vi "Initialize.vi"(7 "Serial Configuration":T1={"Baud Rate"=115200, "Parity"=0, "Data Bits"=8, "Stop Bits"=10, "Flow Control"=0} {"Flow Control" items=["None", "XON/XOFF", "RTS/CTS", "XON/XOFF & RTS/CTS", "DTR/DSR", "XON/XOFF & DTR/DSR"]; "Stop Bits" items=["1.0"=10, "1.5"=15, "2.0"=20]; "Data Bits" items=["7"=7, "8"=8]; "Parity" items=["None", "Odd", "Even", "Mark", "Space"]; "Baud Rate" items=["300"=300, "600"=600, "1200"=1200, "2400"=2400, "4800"=4800, "9600"=9600, "19200"=19200]}, 8 "error in (no error)":errorcluster, 10 "ID Query (True)":bool=TRUE, 11 "VISA resource name":refnum<visa-resource-name>) -> (0 "error out":errorcluster, 3 "VISA resource name out":refnum<visa-resource-name>)   [LabVIEW 2012, in "Roboteq.lvlib"]
doc: "Establishes communication with the sensor and optionally performs a sensor identification query. Therefore, call this VI before calling other sensor driver VIs for this sensor. Generally, you need to call the Initialize VI only once at the beginning of an application."
uses:
  Roboteq.lvlib
panel:
  out "read buffer 2":string
  out "Session Out":refnum<visa-resource-name>
  out "error out 3":errorcluster {"code" format="%.0x"}
  out "token":string
  in  "error in":errorcluster {"code" format="%.0x"}
  in  "Session In":refnum<visa-resource-name>="COM7"
  out "error out 2":errorcluster
  out "read buffer":string
  # "(c) 2010 National Instruments.  ALL RIGHTS RESERVED."
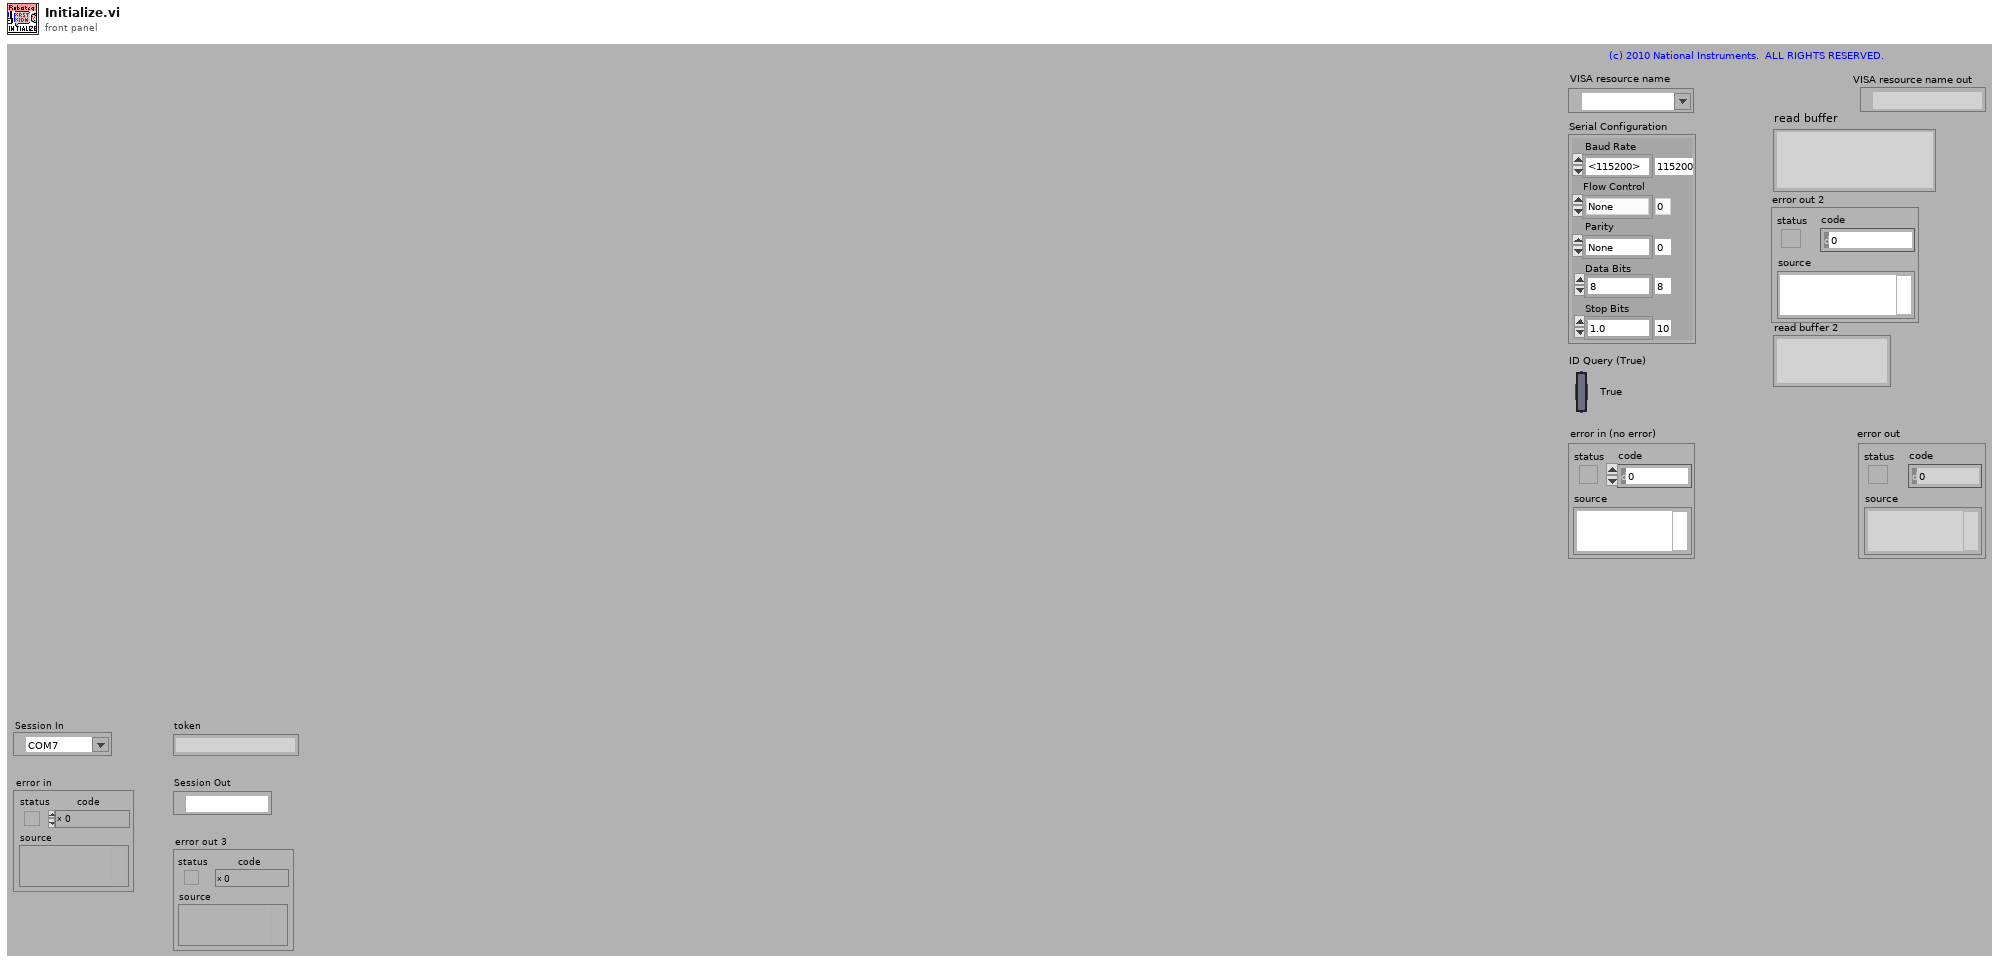
[diagram p1: front panel]
types:
  T1 = cluster{"Baud Rate":u32, "Parity":u16, "Data Bits":u16, "Stop Bits":u16, "Flow Control":u16}
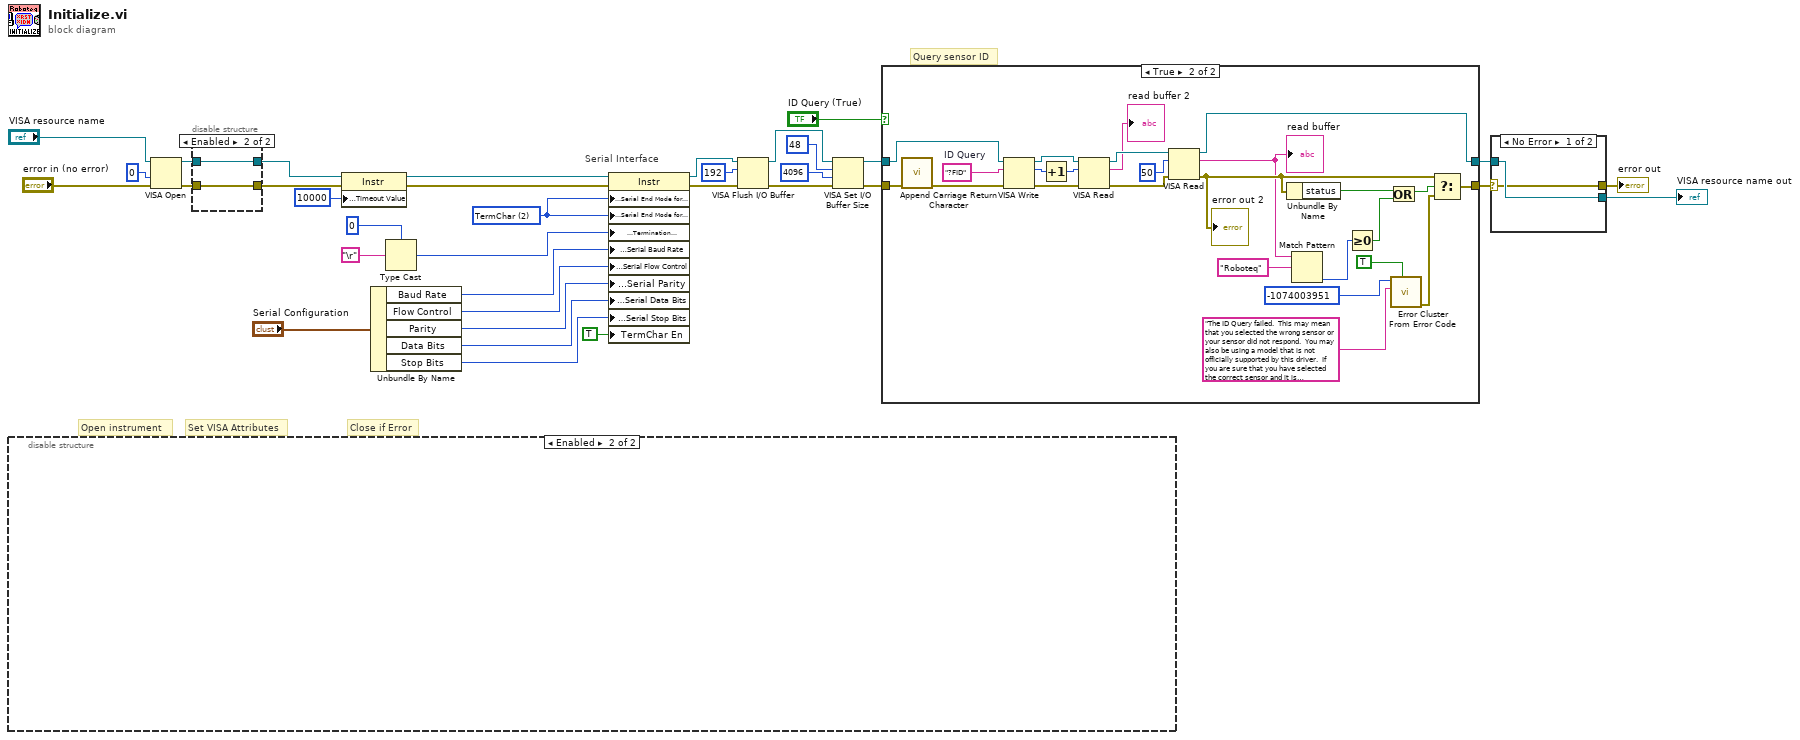
[diagram p0: block diagram]
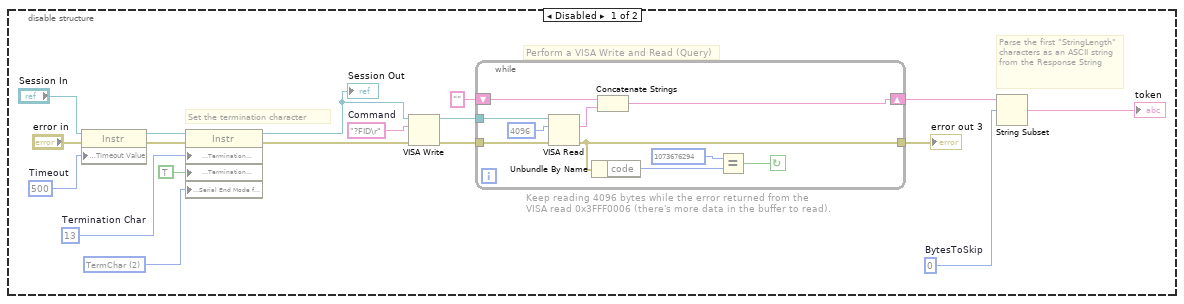
[diagram p2: hidden frame]
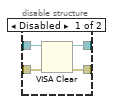
[diagram p3: hidden frame]
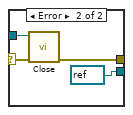
[diagram p4: hidden frame]
diagram:
  w10 = u16 2 items=["None", "LastBit", "TermChar"] ("Serial Settings:Serial End Mode for Reads")
  # "Serial Interface"
  # "Set VISA Attributes"
  # "Close if Error"
  # "Query sensor ID"
  # "Open instrument"
  n1 = disable-structure shown="Enabled" {
    frame Disabled {
      w37 = 0  # BytesToSkip
      w40 = "?FID\r"  # Command
      w45 = u16 2 items=["None", "LastBit", "TermChar"] ("ASRLEndIn")
      w48 = u8 13  # Termination Char
      w53 = u32 500  # Timeout
      # "Parse the first \"StringLength\" characters as an ASCII string from the Response String"
      # "Perform a VISA Write and Read (Query)"
      # "Keep reading 4096 bytes while the error returned from the\nVISA read 0x3FFF0006 (there's more data in the buffer to read)."
      # "Set the termination character"
      n2 = property class="Instr"(reference="Session In", error in="error in", "General Settings:Timeout Value"=w53) -> (reference out=w47:refnum<visa-resource-name>, error out=w50:errorcluster)
      n3 = property class="Instr"(reference=w47, error in=w50, "Message Based Settings:Termination Character"=w48, "Message Based Settings:Termination Character Enable"=TRUE ("enable"), "Serial Settings:Serial End Mode for Reads"=w45) -> (reference out=w36:refnum<visa-resource-name>, error out=w49:errorcluster)
      "Session Out" <- w36
      n4 = VISA Write(VISA resource name=w36, write buffer=w40, error in (no error)=w49) -> (VISA resource name out=w44:refnum<visa-resource-name>, error out=w43:errorcluster)  [unwired: 1 out]
      n5 = while {
        tunnel: w44 -> [w60]
        shift-right: [w54] -> w38
        shift-left: "" -> [w59]
        tunnel: w43 -> [w57]
        tunnel: [w56] -> w42
        stop <- w55 continue-if-true
        n6 = VISA Read(VISA resource name=w60, byte count=u32 4096 ("byte count (0)"), error in (no error)=w57) -> (read buffer=w58:string, error out=w56:errorcluster)  [unwired: 2 out]
        n7 = Unbundle By Name(w56) -> ("code"=w62:i32)
        n8 = Concatenate Strings(w59, w58) -> (w54:string)
        n9 = Equal?(x=1073676294, y=w62) -> (x = y?=w55:bool)
      }
      "error out 3" <- w42
      n10 = String Subset(string=w38, offset (0)=w37) -> (substring=→"token":string)  [unwired: 1 out]
    }
    frame Enabled {
    }
  }
  n11 = VISA Open(access mode=u32 0, error in (no error)="error in (no error)", VISA resource name="VISA resource name") -> (VISA resource name=w26:refnum<visa-resource-name>, error out=w25:errorcluster)  [unwired: 2 in]
  n12 = disable-structure shown="Enabled" {
    disable-tunnel: w26 -> [w67 w69]
    disable-tunnel: w25 -> [w66 w68]
    disable-tunnel: [w65 w69] -> w24
    disable-tunnel: [w64 w68] -> w23
    frame Disabled {
      n13 = VISA Clear(VISA resource name=w67, error in (no error)=w66) -> (VISA resource name out=w65:refnum<visa-resource-name>, error out=w64:errorcluster)
    }
    frame Enabled {
    }
  }
  n14 = property class="Instr"(reference=w24, error in=w23, "General Settings:Timeout Value"=u32 10000) -> (reference out=w29:refnum<visa-resource-name>, error out=w28:errorcluster)
  n15 = Unbundle By Name("Serial Configuration") -> ("Baud Rate"=w8:u32, "Flow Control"=w4:u16, "Parity"=w6:u16, "Data Bits"=w7:u16, "Stop Bits"=w3:u16)
  n16 = Type Cast(type=u8 0, x="\r") -> (*(type *) &x=w9:u8)
  n17 = property class="Instr"(reference=w29, error in=w28, "Serial Settings:Serial End Mode for Reads"=w10, "Serial Settings:Serial End Mode for Writes"=w10, "Message Based Settings:Termination Character"=w9, "Serial Settings:Serial Baud Rate"=w8, "Serial Settings:Serial Flow Control"=w4, "Serial Settings:Serial Parity"=w6, "Serial Settings:Serial Data Bits"=w7, "Serial Settings:Serial Stop Bits"=w3, "TermChar En"=TRUE) -> (reference out=w16:refnum<visa-resource-name>, error out=w18:errorcluster)
  n18 = VISA Flush I/O Buffer(VISA resource name=w16, mask (16)=u16 192, error in (no error)=w18) -> (VISA resource name out=w19:refnum<visa-resource-name>, error out=w17:errorcluster)
  n19 = VISA Set I/O Buffer Size(VISA resource name=w19, mask (16)=u16 48, size (4096)=u32 4096 ("size (0)"), error in (no error)=w17) -> (VISA resource name out=w31:refnum<visa-resource-name>, error out=w30:errorcluster)
  n20 = case shown="True" "ID Query (True)" {
    tunnel: [w70 w96] -> w1
    tunnel: [w71 w82] -> w20
    tunnel: w31 -> [w71 w95]
    tunnel: w30 -> [w70 w85]
    frame False {
    }
    frame True {
      w83 = "?FID"  # ID Query
      n21 = call "Append Carriage Return Character.vi"("error in (no error)"=w85) -> ("error out"=w84:errorcluster)  [unwired: 9 in, 1 out]
      n22 = VISA Write(VISA resource name=w95, write buffer=w83, error in (no error)=w84) -> (VISA resource name out=w76:refnum<visa-resource-name>, return count=w75:u32, error out=w74:errorcluster)
      n23 = Increment(x=w75) -> (x+1=w72:u32)
      n24 = VISA Read(VISA resource name=w76, byte count=w72, error in (no error)=w74) -> (VISA resource name out=w80:refnum<visa-resource-name>, read buffer=→"read buffer 2":string, error out=w79:errorcluster)  [unwired: 1 out]
      n25 = VISA Read(VISA resource name=w80, byte count=u32 50, error in (no error)=w79) -> (VISA resource name out=w82:refnum<visa-resource-name>, read buffer=w78:string, error out=w81:errorcluster)  [unwired: 1 out]
      "read buffer" <- w78
      "error out 2" <- w81
      n26 = Unbundle By Name(w81) -> ("status"=w88:bool)
      n27 = Match Pattern(string=w78, regular expression="Roboteq") -> (offset past match=w89:i32)  [unwired: 1 in, 3 out]
      n28 = Greater Or Equal To 0?(x=w89) -> (x >= 0?=w87:bool)
      n29 = Or(x=w88, y=w87) -> (x .or. y?=w86:bool)
      n30 = call <vilib>:"Error Cluster From Error Code.vi"("show call chain? (False)"=TRUE, "error message (\"\")"="The ID Query failed.  This may mean that you selected the wrong sensor or your sensor did not respond.  You may also be using a model that is not officially supported by this driver.  If you are sure that you have selected the correct sensor and it is responding, try disabling the ID Query." ("Source (VI Name)"), "error code (0)"=-1074003951 ("Code")) -> ("error out"=w93:errorcluster)  [unwired: 6 in]
      n31 = Select(t=w81, s=w86, f=w93) -> (s? t:f=w96:errorcluster)
    }
  }
  n32 = case shown="No Error" w1 {
    selector: w1 -> [w97 w100]
    tunnel: w20 -> [w98 w101]
    tunnel: [w98 refnum<visa-resource-name> refnum ("VISA resource name out")] -> w22
    tunnel: [w97 w102] -> w21
    frame No Error {
    }
    frame Error {
      n33 = call "Close.vi"("error in (no error)"=w100, "VISA resource name"=w101) -> ("error out"=w102:errorcluster)  [unwired: 9 in]
    }
  }
  "VISA resource name out" <- w22
  "error out" <- w21
